vi "2Voice.FrameReader.vi"(5 "写入参数":string, 6 "Return Length":u8, 7 "timeout (10sec)":u32=3000 caption="超时（10秒）", 8 "error in (no error)":errorcluster caption="错误输入（无错误）", 9 "Para":u8[](array[numeric]) format="%02x", 10 "Frame CMD":T1(ring), 11 "FrameReader Port":refnum<visa-resource-name> caption="VISA资源名称") -> (0 "错误输出":errorcluster, 1 "写入命令":u8[](array[numeric]) format="%02x", 2 "读取缓冲区":string, 3 "OK?":bool, 4 "return":u8[](array[numeric]) format="%02x")   [LabVIEW 2012, in "Lib_UEL.ATE.lvlib" / "Lib_2Voice.lvlib"]
uses:
  Lib_2Voice.lvlib
  <vilib>/Instr/_visa.llb/VISA Configure Serial Port (Instr).vi
  App/Lib_App.lvlib
panel:
  out "命令输出(字符串)":string
  # "2012-08-20: OpenAudio命令没有返回值，但必须等待返回才能生效，设置返回字节数为1即可。\n 2012-09-13: \n - 增加带参数的呼叫命令 \n - 增加返回值长度的参数，至少都读取一个字节的返回值\n 2012-10-06\n - 增加自定义命令发送\n 2015-11-03\n - 增加写入参数的文本输入.80 00 CB FF A5 5A FF A5 5A 54 45 53 54 99 81"
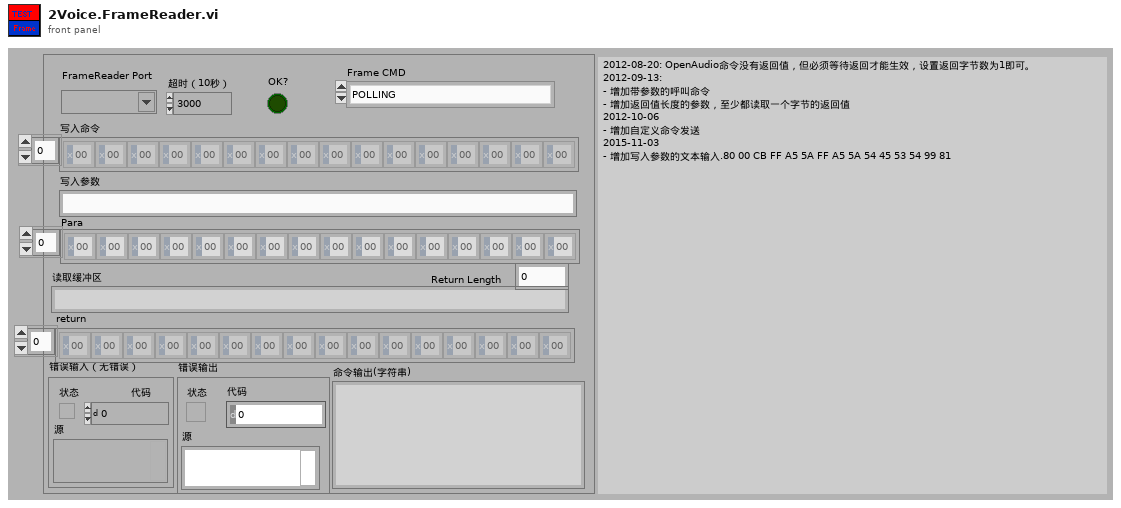
[diagram p1: front panel]
types:
  T1 = enum16{"POLLING", "CHIAMATA", "TEST_DRIVER", "ENTER_TEST_MODE", "CHIAMATA4AudioSetting", "CHIAMATA.FF", "POLLING.FF", "TEST(For BTWIN)", "TestFrame(BTWIN)", "CHIAMATA.7F", "STATO_PORTA_ISTANTANEO", "CHIAMATA.Video", "CHIAMATA.Video.FF", "STATO_PORTA_ISTANTANEO_OFF", "TestFrame_Data_02", "ACK PANICO", "LINEA LIBERA", "TestFrame_Data_03", "CallAudio From 2nd VPE(0x7F)", "Auto Insertion", "Open Audio", "AP2 Command", "CallFrame as 2nd Family VPE", "DEBUG FRAME-01", "DEBUG FRAME-03", "SELF Insertion", "CHIAMATA_Para", "Def_CMD"}
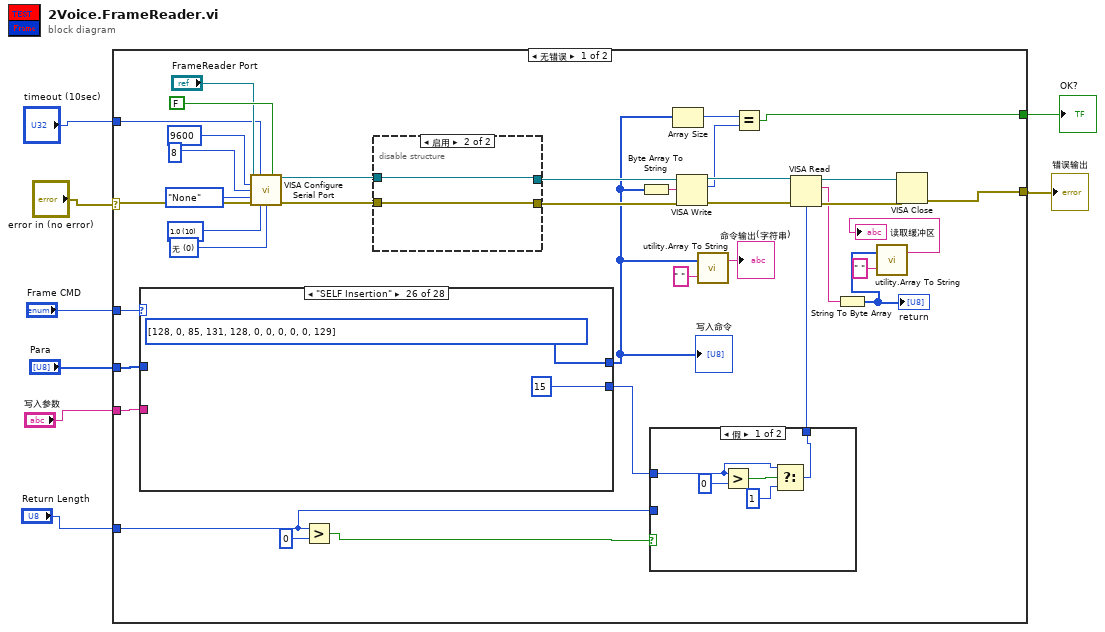
[diagram p0: block diagram]
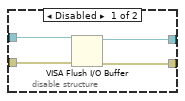
[diagram p3: hidden frame]
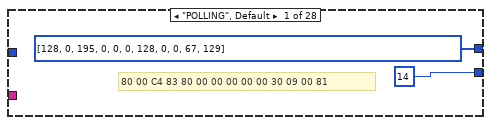
[diagram p4: hidden frame]
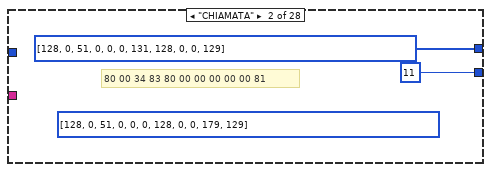
[diagram p5: hidden frame]
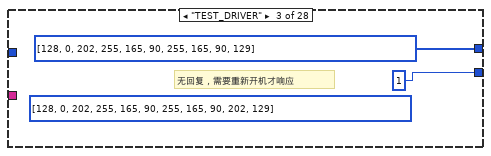
[diagram p6: hidden frame]
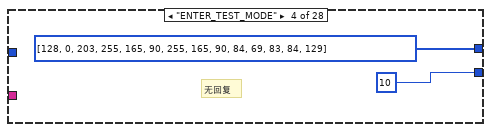
[diagram p7: hidden frame]
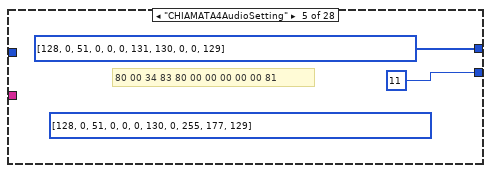
[diagram p8: hidden frame]
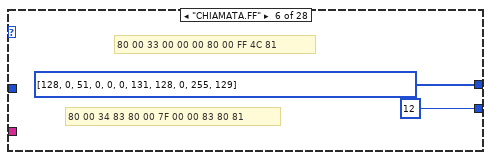
[diagram p9: hidden frame]
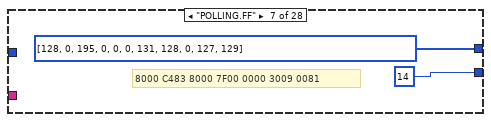
[diagram p10: hidden frame]
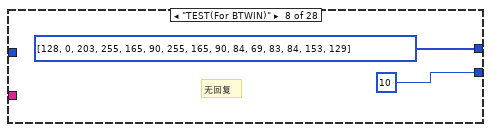
[diagram p11: hidden frame]
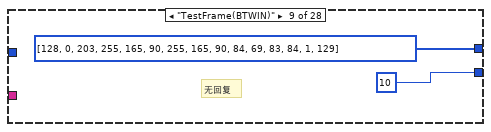
[diagram p12: hidden frame]
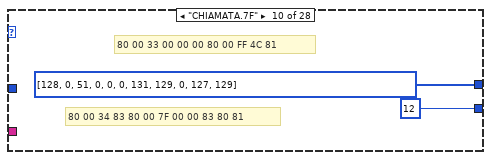
[diagram p13: hidden frame]
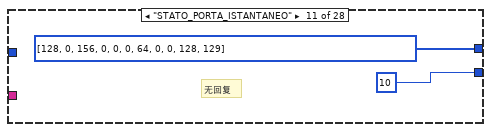
[diagram p14: hidden frame]
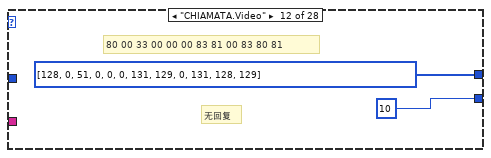
[diagram p15: hidden frame]
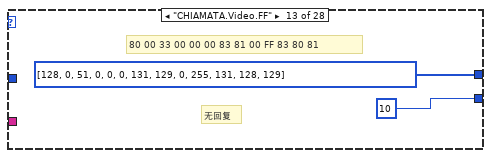
[diagram p16: hidden frame]
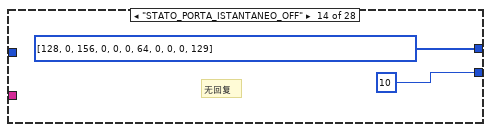
[diagram p17: hidden frame]
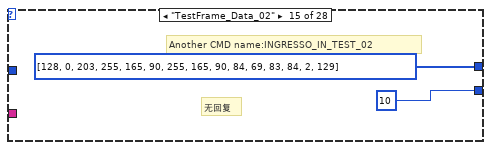
[diagram p18: hidden frame]
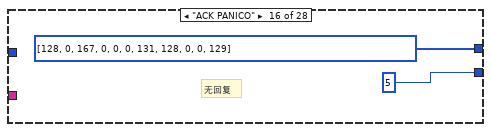
[diagram p19: hidden frame]
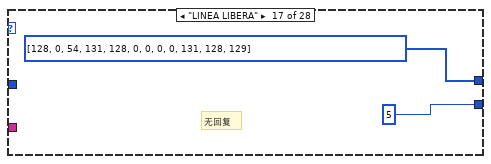
[diagram p20: hidden frame]
diagram:
  n1 = case shown="无错误" "error in (no error)" {
    selector: "error in (no error)" -> [w37 w134]
    tunnel: "Frame CMD" -> [w38 _]
    tunnel: [w31 w134] -> w6
    tunnel: "timeout (10sec)" -> [w30 _]
    tunnel: [w23 FALSE] -> w4
    tunnel: "Para" -> [w22 _]
    tunnel: "Return Length" -> [w18 _]
    tunnel: "写入参数" -> [w9 _]
    frame No Error {
      w45 = u16 0 items=["无", "XON/XOFF", "RTS/CTS", "XON/XOFF & RTS/CTS", "DTR/DSR", "XON/XOFF & DTR/DSR"] ("flow control (0:none)")
      w44 = u16 10 items=["1.0"=10, "1.5"=15, "2.0"=20] ("stop bits (10: 1 bit)")
      n2 = case shown="\"SELF Insertion\"" w38 {
        tunnel: [u8[] [128, 0, 195, 0, 0, 0, 128, 0, 0, 67, 129] ("无符号字节数组") u8[] [128, 0, 51, 0, 0, 0, 131, 128, 0, 0, 129] ("无符号字节数组") u8[] [128, 0, 202, 255, 165, 90, 255, 165, 90, 129] ("无符号字节数组") u8[] [128, 0, 203, 255, 165, 90, 255, 165, 90, 84, 69, 83, 84, 129] ("无符号字节数组") u8[] [128, 0, 51, 0, 0, 0, 131, 130, 0, 0, 129] ("无符号字节数组") u8[] [128, 0, 51, 0, 0, 0, 131, 128, 0, 255, 129] ("无符号字节数组") u8[] [128, 0, 195, 0, 0, 0, 131, 128, 0, 127, 129] ("无符号字节数组") u8[] [128, 0, 203, 255, 165, 90, 255, 165, 90, 84, 69, 83, 84, 153, 129] ("无符号字节数组") u8[] [128, 0, 203, 255, 165, 90, 255, 165, 90, 84, 69, 83, 84, 1, 129] ("无符号字节数组") u8[] [128, 0, 51, 0, 0, 0, 131, 129, 0, 127, 129] ("无符号字节数组") u8[] [128, 0, 156, 0, 0, 0, 64, 0, 0, 128, 129] ("无符号字节数组") u8[] [128, 0, 51, 0, 0, 0, 131, 129, 0, 131, 128, 129] ("无符号字节数组") u8[] [128, 0, 51, 0, 0, 0, 131, 129, 0, 255, 131, 128, 129] ("无符号字节数组") u8[] [128, 0, 156, 0, 0, 0, 64, 0, 0, 0, 129] ("无符号字节数组") u8[] [128, 0, 203, 255, 165, 90, 255, 165, 90, 84, 69, 83, 84, 2, 129] ("无符号字节数组") u8[] [128, 0, 167, 0, 0, 0, 131, 128, 0, 0, 129] ("无符号字节数组") u8[] [128, 0, 54, 131, 128, 0, 0, 0, 0, 131, 128, 129] ("无符号字节数组") u8[] [128, 0, 203, 255, 165, 90, 255, 165, 90, 84, 69, 83, 84, 3, 129] ("无符号字节数组") u8[] [128, 0, 51, 32, 0, 0, 131, 128, 0, 127, 129] ("无符号字节数组") u8[] [128, 0, 85, 128, 0, 131, 17, 0, 0, 0, 129] ("无符号字节数组") u8[] [128, 0, 53, 128, 0, 131, 17, 0, 0, 0, 129] ("无符号字节数组") u8[] [128, 0, 57, 131, 128, 0, 0, 0, 0, 0, 129] ("无符号字节数组") u8[] [128, 0, 51, 0, 0, 1, 131, 128, 0, 0, 129] ("无符号字节数组") u8[] [128, 0, 208, 64, 0, 0, 131, 128, 3, 1, 129] ("无符号字节数组") u8[] [128, 0, 208, 64, 0, 0, 131, 128, 0, 0, 129] ("无符号字节数组") u8[] [128, 0, 85, 131, 128, 0, 0, 0, 0, 0, 129] ("无符号字节数组") w110 w122] -> w15
        tunnel: [14 ("y") 11 1 ("y") 10 ("y") 11 12 14 ("y") 10 ("y") 10 ("y") 12 10 ("y") 10 ("y") 10 ("y") 10 ("y") 10 ("y") 5 ("y") 5 ("y") 10 ("y") 11 17 1 15 11 15 15 15 24 w127] -> w17
        tunnel: w22 -> [_ _ _ _ _ _ _ _ _ _ _ _ _ _ _ _ _ _ _ _ _ _ _ _ _ _ w115 w123]
        tunnel: w9 -> [_ _ _ _ _ _ _ _ _ _ _ _ _ _ _ _ _ _ _ _ _ _ _ _ _ _ _ w121]
        frame "POLLING", Default {
          # "80 00 C4 83 80 00 00 00 00 00 30 09 00 81"
        }
        frame "CHIAMATA" {
          (unwired) u8[] [128, 0, 51, 0, 0, 0, 128, 0, 0, 179, 129] ("无符号字节数组")
          # "80 00 34 83 80 00 00 00 00 00 81"
        }
        frame "TEST_DRIVER" {
          (unwired) u8[] [128, 0, 202, 255, 165, 90, 255, 165, 90, 202, 129] ("无符号字节数组")
          # "无回复，需要重新开机才响应"
        }
        frame "ENTER_TEST_MODE" {
          # "无回复"
        }
        frame "CHIAMATA4AudioSetting" {
          (unwired) u8[] [128, 0, 51, 0, 0, 0, 130, 0, 255, 177, 129] ("无符号字节数组")
          # "80 00 34 83 80 00 00 00 00 00 81"
        }
        frame "CHIAMATA.FF" {
          # "80 00 34 83 80 00 7F 00 00 83 80 81"
          # "80 00 33 00 00 00 80 00 FF 4C 81"
        }
        frame "POLLING.FF" {
          # "8000 C483 8000 7F00 0000 3009 0081"
        }
        frame "TEST(For BTWIN)" {
          # "无回复"
        }
        frame "TestFrame(BTWIN)" {
          # "无回复"
        }
        frame "CHIAMATA.7F" {
          # "80 00 34 83 80 00 7F 00 00 83 80 81"
          # "80 00 33 00 00 00 80 00 FF 4C 81"
        }
        frame "STATO_PORTA_ISTANTANEO" {
          # "无回复"
        }
        frame "CHIAMATA.Video" {
          # "80 00 33 00 00 00 83 81 00 83 80 81"
          # "无回复"
        }
        frame "CHIAMATA.Video.FF" {
          # "80 00 33 00 00 00 83 81 00 FF 83 80 81"
          # "无回复"
        }
        frame "STATO_PORTA_ISTANTANEO_OFF" {
          # "无回复"
        }
        frame "TestFrame_Data_02" {
          # "Another CMD name:INGRESSO_IN_TEST_02"
          # "无回复"
        }
        frame "ACK PANICO" {
          # "无回复"
        }
        frame "LINEA LIBERA" {
          # "无回复"
        }
        frame "TestFrame_Data_03" {
          # "无回复"
        }
        frame "CallAudio From 2nd VPE(0x7F)" {
          # "返回: 80 00 34 83 80 00 7F 30 00 00 81"
          # "80 00 33 20 00 00 83 80 00 7F 81"
        }
        frame "Auto Insertion" {
          # "80 00 56 00 00 00 83 80 00 11 00 81 80 00 5A 01 81"
          # "返回: 80 00 56 00 00 00 83 80 00 11 00 81 80 00 5A 01 81"
          # "80 00 55 80 00 83 11 00 00 00 81"
        }
        frame "Open Audio" {
          # "Another name: UNHOOK"
          # "80 00 35 80 00 83 11 00 00 00 81"
          # "80 00 35 80 00 83 11 00 00 00 81"
        }
        frame "AP2 Command" {
          # "返回: 8000 3A00 0000 4000 0082 8380 0000 81"
          # "80 00 39 83 80 00 00 00 00 00 81"
        }
        frame "CallFrame as 2nd Family VPE" {
          # "返回: 80 00 34 83 80 00 00 10 00 01 81"
          # "80 00 33 00 00 01 83 80 00 00 81"
        }
        frame "DEBUG FRAME-01" {
        }
        frame "DEBUG FRAME-03" {
        }
        frame "SELF Insertion" {
        }
        frame "CHIAMATA_Para" {
          n3 = Index Array(array=w115, index=0 ("索引")) -> (element=w117:u8)
          n4 = Array Subset(array=w115, index=1 ("索引"), length=u8 2 ("新元素/子数组")) -> (w112:u8[])
          n5 = Build Array (concatenate)(u8[] [128, 0, 51] ("无符号字节数组"), w117, u8[] [0, 0, 131, 129] ("无符号字节数组"), w112, u8[] [129] ("无符号字节数组")) -> (w110:u8[])
        }
        frame "Def_CMD" {
          n6 = String Length(string=w121) -> (length=w126:i32)
          n7 = Greater?(x=w126, y=0) -> (0:w124:bool)
          n8 = case shown="真" w124 {
            tunnel: [24 24] -> w127
            tunnel: w123 -> [w129 _]
            tunnel: [w129 w130] -> w122
            tunnel: w121 -> [_ w131]
            frame False {
            }
            frame True {
              n9 = call "utility.String to Array.vi"("命令输入"=w131) -> ("输出数组"=w130:u8[])
            }
          }
        }
      }
      "写入命令" <- w15
      n10 = call-poly "VISA Configure Serial Port"("VISA resource name"="FrameReader Port", "timeout (10sec)"=w30, "Enable Termination\nChar (T)"=FALSE ("Disable Termination\nChar (T)"), "baud rate (9600)"=u32 9600, "data bits (8)"=u16 8, "parity (0:none)"=enum16{"None", "Odd", "Even", "Mark", "Space"}."None", "error in (no error)"=w37, "stop bits (10: 1 bit)"=w44, "flow control (0:none)"=w45) -> ("VISA resource name out"=w29:refnum<visa-resource-name>, "error out"=w28:errorcluster)  [unwired: 5 in]
      n11 = Greater?(x=w18, y=u8 0) -> (0:w20:bool)
      n12 = disable-structure shown="启用" {
        disable-tunnel: w29 -> [w55 w57]
        disable-tunnel: w28 -> [w54 w56]
        disable-tunnel: [w53 w57] -> w27
        disable-tunnel: [w52 w56] -> w26
        frame Disabled {
          n13 = VISA Flush I/O Buffer(VISA resource name=w55, error in (no error)=w54) -> (VISA resource name out=w53:refnum<visa-resource-name>, error out=w52:errorcluster)  [unwired: 1 in]
        }
        frame Enabled {
        }
      }
      n14 = Byte Array To String(unsigned byte array=w15) -> (string=w36:string)
      n15 = case shown="假" w20 {
        tunnel: [w46 w51] -> w19
        tunnel: w18 -> [_ w51]
        tunnel: w17 -> [w48 _]
        frame False {
          n16 = Greater?(x=w48, y=0) -> (0:w49:bool)
          n17 = Select(t=w48, s=w49, f=1 ("y")) -> (s? t:f=w46:i32)
        }
        frame True {
        }
      }
      n18 = Array Size(array=w15) -> (size(s)=w25:i32)
      n19 = VISA Write(VISA resource name=w27, write buffer=w36, error in (no error)=w26) -> (VISA resource name out=w34:refnum<visa-resource-name>, return count=w24:u32, error out=w35:errorcluster)
      n20 = call "utility.Array To String.vi"("分隔符输入"=" ", "无符号字节数组"=w15) -> ("命令输出(字符串)"=→"命令输出(字符串)":string)  [unwired: 1 out]
      n21 = Equal?(x=w25, y=w24) -> (x = y?=w23:bool)
      n22 = VISA Read(VISA resource name=w34, byte count=w19, error in (no error)=w35) -> (VISA resource name out=w33:refnum<visa-resource-name>, read buffer=w16:string, error out=w32:errorcluster)  [unwired: 1 out]
      n23 = String To Byte Array(string=w16) -> (unsigned byte array=w10:u8[])
      "return" <- w10
      n24 = call "utility.Array To String.vi"("分隔符输入"=" ", "无符号字节数组"=w10) -> ("命令输出(字符串)"=→"读取缓冲区":string)  [unwired: 1 out]
      n25 = VISA Close(VISA resource name=w33, error in (no error)=w32) -> (error out=w31:errorcluster)
    }
    frame Error {
    }
  }
  "错误输出" <- w6
  "OK?" <- w4
